vi "Inline - Reset Acyclic Labels Trigger Channels.vi"(8 "error in (no error)":errorcluster, 11 "Inline Status Channels Refs":T1[](array[typedef]) format="%.0x") -> (0 "error out":errorcluster)   [LabVIEW 2019, in "Ballard Arinc-429 Engine.lvlib"]
uses:
  Ballard Arinc-429 Engine.lvlib
  <vilib>/NI VeriStand/Custom Device API/Data Reference.ctl
  <vilib>/NI VeriStand/Custom Device API/Custom Device API.lvlib
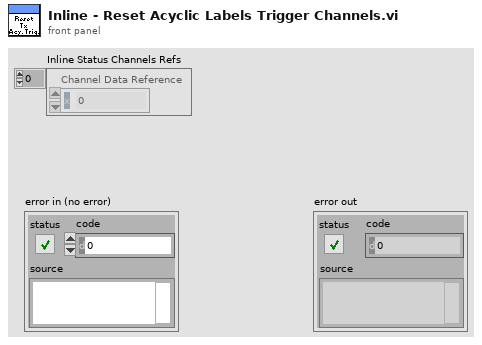
[diagram p1: front panel]
types:
  T1 = typedef "Custom Device API.lvlib/Data Reference.ctl" = i32
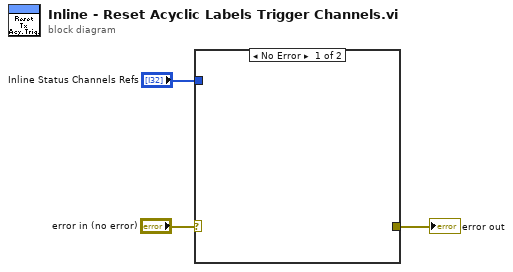
[diagram p0: block diagram]
diagram:
  n1 = case shown="No Error" "error in (no error)" {
    selector: "error in (no error)" -> [_ w4]
    tunnel: [_ w4] -> w2
    tunnel: "Inline Status Channels Refs" -> [_ _]
    frame No Error {
    }
    frame Error {
    }
  }
  "error out" <- w2
